vi "set Baud Rate.vi"(8 "error in (no error)":errorcluster, 10 "baudrate":i32, 11 "port_num":i32) -> (0 "error out":errorcluster, 3 "function return":u8)   [LabVIEW 2018, in "labview.lvlib"]
doc: "WINDECLSPEC uint8_t setBaudRate (int port_num, const int baudrate);"
uses:
  labview.lvlib
  dxl_x86_c.dll
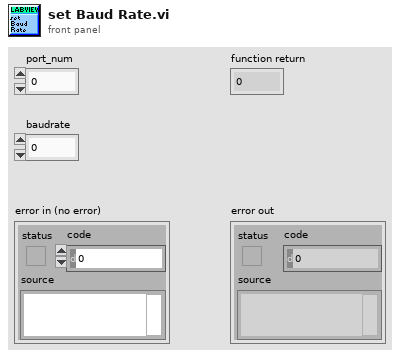
[diagram p1: front panel]
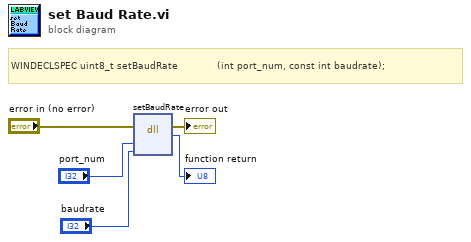
[diagram p0: block diagram]
diagram:
  # "WINDECLSPEC uint8_t setBaudRate             (int port_num, const int baudrate);"
  n1 = dll-call lib="C:/Users/joaos/OneDrive/Documents/[PhD]/Project Omnidirectional Vehicle/Vanes/LabView_code/joaoandthethreestands/DynamixelSDK-3.7.31/labview/new_compilation/dxl_x86_c.*" fn="setBaudRate"(error in="error in (no error)", "port_num"="port_num", "baudrate"="baudrate") -> (error out=→"error out":errorcluster, →"function return":u8)  [unwired: 4 in, 1 out]
